vi "Write Status Source.vi"(8 "error in (no error)":errorcluster, 10 "Status Source":T1, 11 "Session in":refnum<class "Session.lvclass">) -> (0 "error out":errorcluster, 3 "Session out":refnum<class "Session.lvclass">)   [LabVIEW 2024, in "CTI.lvlib" / "Session.lvclass"]
doc: "Sets the configuration for when a device's status LED will be lit.\n\n<b>Comms</b> - Lights up the LED for short durations while the device is being interacted with from a host system.\n<b>User</b> - Puts the status LED under control of the software running on the host. Use <b>Write User Status.vi</b> to set whether the LED is lit or not while in User source mode."
uses:
  Session.lvclass
  Status Source.ctl
  DeviceComms/DeviceComms.lvclass
  CTI.lvlib
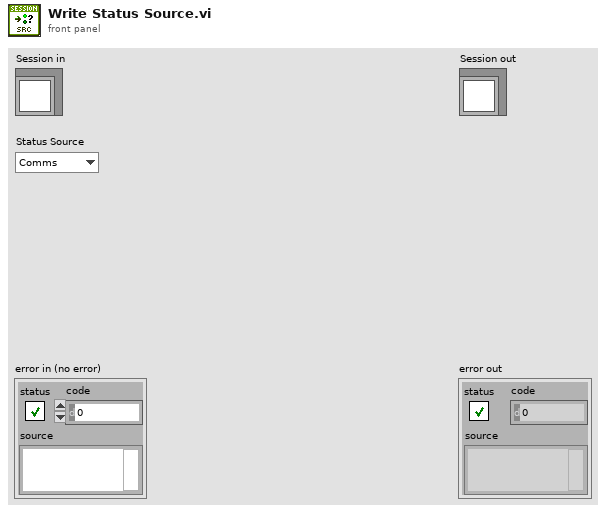
[diagram p1: front panel]
types:
  T1 = typedef "CTI.lvlib/Status Source.ctl" = enum16{"Comms", "User"}
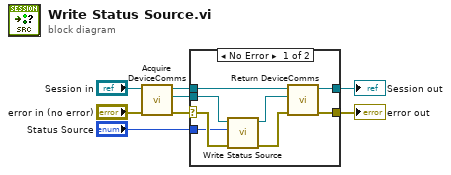
[diagram p0: block diagram]
diagram:
  n1 = call "Acquire DeviceComms.vi"("error in (no error)"="error in (no error)", "Session in"="Session in") -> ("error out"=w8:errorcluster, "DeviceComms"=w4:refnum<class "DeviceComms.lvclass">, "Session out"=w5:refnum<class "Session.lvclass">)  [unwired: 7 in]
  n2 = case shown="No Error" w8 {
    selector: w8 -> [w16 w17]
    tunnel: w5 -> [w15 w18]
    tunnel: w4 -> [w14 _]
    tunnel: "Status Source" -> [w13 _]
    tunnel: [w12 w18] -> w2
    tunnel: [w9 w17] -> w1
    frame No Error {
      n3 = call-dynamic "Write Status Source.vi"("error in (no error)"=w16, "Status Source"=w13, "DeviceComms in"=w14) -> ("error out"=w10:errorcluster, "DeviceComms out"=w11:refnum<class "DeviceComms.lvclass">)  [unwired: 7 in]
      n4 = call "Return DeviceComms.vi"("error in (no error)"=w10, "DeviceComms"=w11, "Session in"=w15) -> ("error out"=w9:errorcluster, "Session out"=w12:refnum<class "Session.lvclass">)  [unwired: 7 in]
    }
    frame Error {
    }
  }
  "error out" <- w1
  "Session out" <- w2
